vi "LCDIO Write On.vi"(7 "On":bool, 8 "error in (no error)":errorcluster caption="Fehler (Eingang, kein Fehler)", 11 "Output Channel Handle":i64) -> (0 "error out":errorcluster caption="Fehler (Ausgang)")   [LabVIEW 2021, in "labbCAN_DigIO_API.lvlib"]
doc: "LCDIO_Func long LCDIO_CALL LCDIO_WriteOn(dev_hdl OutChanHdl, unsigned char On);"
uses:
  labbCAN_DigIO_API.lvlib
  labbCAN_DigIO_API.dll
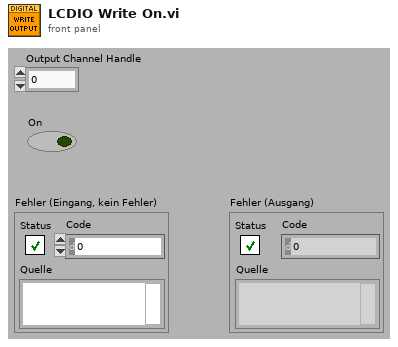
[diagram p1: front panel]
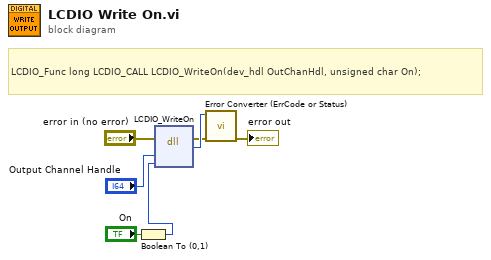
[diagram p0: block diagram]
diagram:
  # "LCDIO_Func long LCDIO_CALL LCDIO_WriteOn(dev_hdl OutChanHdl, unsigned char On);"
  n1 = Boolean To (0,1)(Boolean="On") -> (0, 1=w1:i16)
  n2 = dll-call lib="C:/Users/olaja/AppData/Local/CETONI_SDK/labbCAN_DigIO_API.*" fn="LCDIO_WriteOn"(error in="error in (no error)", "Output Channel Handle"="Output Channel Handle", "On"=w1) -> (error out=w4:errorcluster, "Rückgabetyp"=w5:i32)  [unwired: 4 in, 1 out]
  n3 = call "Error Converter (ErrCode or Status).vi"("error in (no error)"=w4, "error code"=w5) -> ("error out"=→"error out":errorcluster)  [unwired: 9 in]
